vi "Main.vi"() -> ()   [LabVIEW 2022 SP3]
doc: "This Continuous Measurement sample project is based on the Queued Message Handler template.\n\nThe Event Handling Loop generates messages based on user interface actions.\n\nThe Message Handling Loop processes messages generated by the Event Handling Loop, or by other messages. There are also Acquisition and Logging message handling loop subVIs, and a chart updating loop."
uses:
  controls/UI State.ctl
  Settings/Settings.ctl
  Acquisition/Hardware Configuration.ctl
  Logging/Logging Configuration.ctl
  controls/UI Data.ctl
  <vilib>/Utility/miscctls.llb/LVMinMaxIncTypeDef.ctl
  <vilib>/Platform/browser.llb/Open URL in Default Browser (string).vi
  support/Message Queue/Enqueue Message (Array).vi
  <vilib>/Utility/error.llb/Error Cluster From Error Code.vi
  <vilib>/ErrorRing/Error Ring.xnode
  Acquisition/Acquisition.lvlib
  Logging/Logging.lvlib
  Settings/Settings.lvlib
  support/User Event - Stop/User Event - Stop.lvlib
  support/Message Queue/Message Queue.lvlib
  <instrlib>/BK Precision 911X Series/BK Precision 911X Series.lvlib
  Settings/Settings Dialog.vi
  Settings/Logging Settings Dialog.vi
  Settings/PS Settings Dialog.vi
  About.vi
panel:
  out "UI State":T1
  out "List CtlRef":refnum<vi>
  out "Settings CtlRef":refnum<vi>
  out "Output Ref":refnum<vi>
  in  "Clear":bool
  out "Stop":i32
  out "Power":dbl format="%.3g"
  out "Current":dbl format="%.3g"
  out "Voltage":dbl format="%.3g"
  out "model":string
  in  "PS Settings":bool
  in  "Tab Control":enum32{"Monitoring", "List", "Ext.Program"}(tab)
  out "Voltage":dbl(graph)
  out "Power":dbl(graph)
  out "Current":dbl(graph)
  in  "Keep Output Enable":bool
  in  "Enable Logging":bool
  in  "Abort List":bool
  in  "Run List":bool
  in  "List Array":T2(array[cluster]) {"Voltage" min=0.0 max=150.0 step=1.0 format="%.3g"; "Slope" min=0.0 max=30.0 step=1.0 format="%.3g"; "Current" format="%.3g"; "Width" min=0.001 max=86400.0 step=1.0 format="%.3g"}
  in  "List Number":i32=1
  in  "Sequence Number":dbl=1.0
  in  "Save List to PS":bool
  in  "Load List from PS":bool
  in  "List Power Limit":dbl
  in  "Sequence Repeat Count":i32[](array[numeric])
  in  "Linked Sequences":bool[](array[boolean])
  in  "Save Sequence to PS":bool
  in  "Load Sequence from PS":bool
  in  "List Repeat":i32=1 min=1 max=65535 step=1
  in  "Active Steps":bool[](array[boolean])
  out "Delay Time":dbl caption="Elapsed Time (s)"
  out "Elapsed Time (s)":dbl
  out "Start Time":string
  out "Stop Time":string
  out "Current Step":i32
  out "Remaining Steps":i32
  in  "Ext. List Abort":bool
  in  "Ext. List Start":bool
  in  "List Repeat":i32=1 min=1 step=1
  in  "Ext. List Array":T3(array[cluster]) {"Ext. List Voltage" min=0.0 max=150.0 step=1.0 format="%.3g"; "Ext. List Current" min=0.0 max=30.0 step=1.0 format="%.3g"; "Ext. List Time" min=0.001 max=86400.0 format="%.3g"}
  in  "Log Settings":bool
  in  "Meas Out":T4={"Voltage"=0.0, "Current"=0.0, "Power"=0.0, timestamp(3748437232.444618 s since 1904-01-01)}
  in  "Disconnect":bool
  in  "Output Control":bool
  out "ID":string="BK PRECISION, BK9116, 602078010687320001, 0.05-0.02\n"
  in  "Connect":bool
  in  "Inst. Settings":bool
  in  "Current":dbl(knob) min=0.0 max=30.0 step=1.0 scale=0.0..30.0 scale format="%#_3p"
  in  "Voltage":dbl(knob) min=0.0 max=150.0 step=1.0 scale=0.0..150.0 scale format="%#_2p"
  in  "Start":bool
  in  "Stop":bool
  out "Status":string="Exit"
  in  "Exit":bool
  # "Sequence Setup"
  # "List Setup"
  # "Step \nIndex"
  # "Voltage (V)"
  # "Current (A)"
  # "Time (s)"
  # "Output"
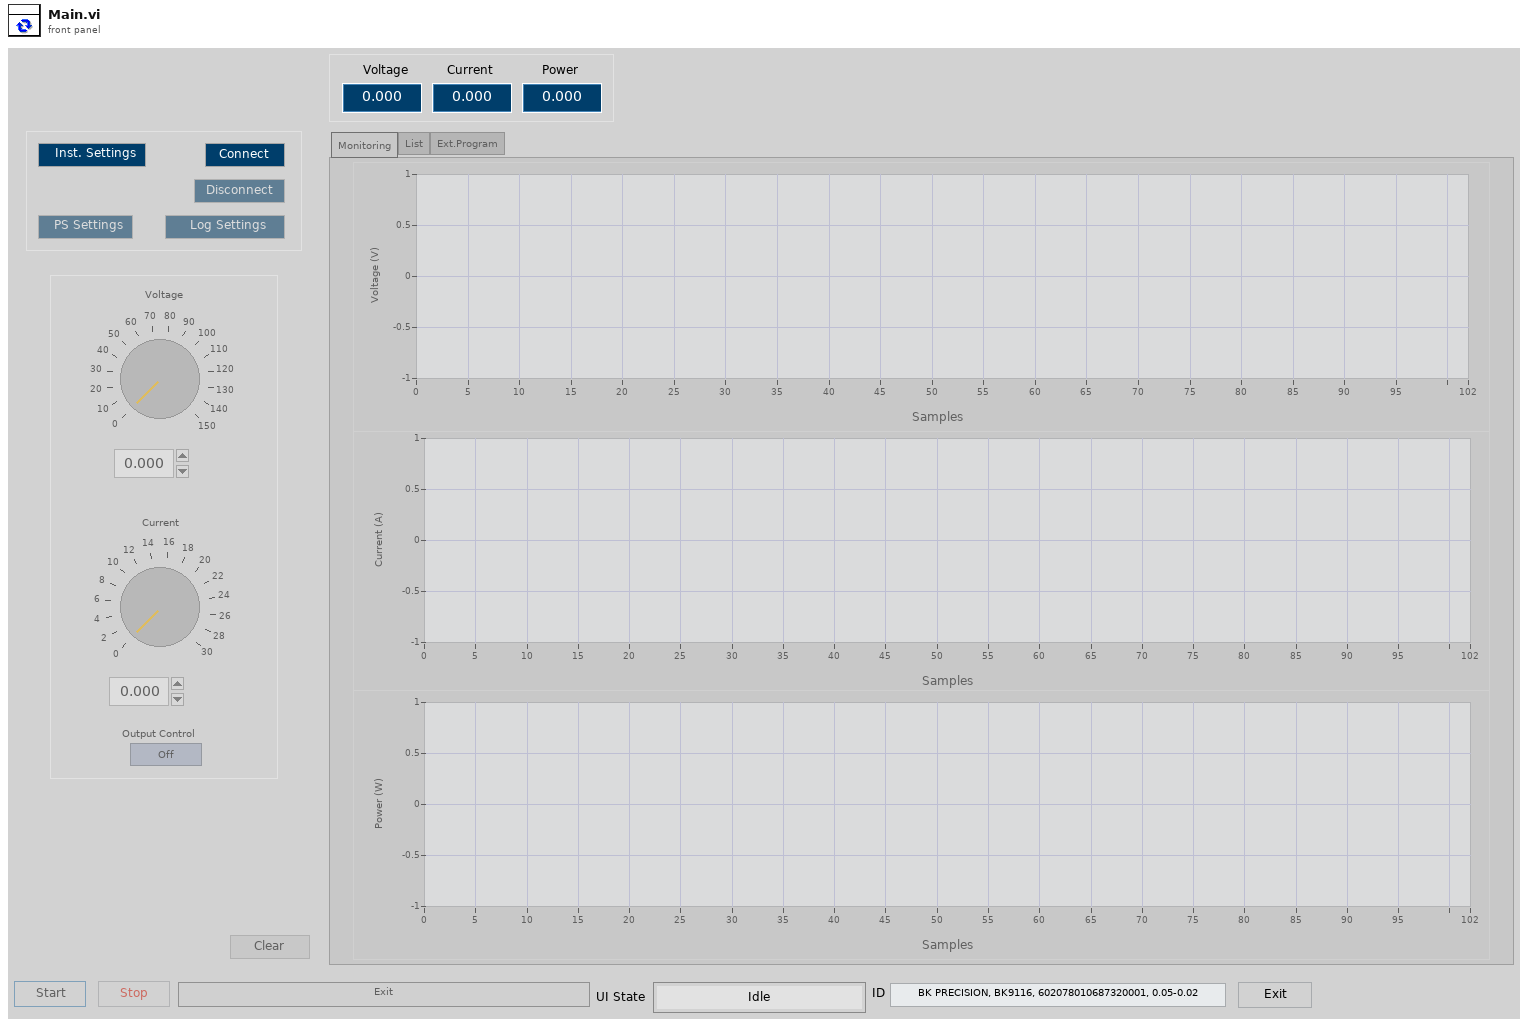
[diagram p1: front panel]
types:
  T1 = typedef "UI State.ctl" = enum16{"Idle", "Acquiring and Logging", "Waiting for Exit", "Waiting for Exit (Acq Stopped)", "Waiting for Exit (Log Stopped)", "Waiting for Stop", "Waiting for Stop (Acq Stopped)", "Waiting for Stop (Log Stopped)"}
  T2 = cluster{"Width":dbl, "Current":dbl, "Slope":dbl, "Voltage":dbl}[]
  T3 = cluster{"Boolean":bool, "Ext. List Time":dbl, "Ext. List Current":dbl, "Ext. List Voltage ":dbl}[]
  T4 = cluster{"Voltage":dbl, "Current":dbl, "Power":dbl, timestamp}
  T5 = cluster{"List Stop COND":i32, "Voltage":dbl, "Current":dbl, "Power":dbl}
  T6 = typedef "UI Data.ctl" = cluster{"Start Ref":refnum<vi>, "Stop Ref":refnum<vi>, "Connect Ref":refnum<vi>, "Exit Ref":refnum<vi>, "Status Ref":refnum<vi>, "Voltage":refnum<vi>, "Current":refnum<vi>, "Output Control":refnum<vi>, "TabCtl Refnum":refnum<vi>, "Inst.Settings Refnum":refnum<vi>, "PS Settings Refnum":refnum<vi>, "Log Settings Refnum":refnum<vi>, "Clear Refnum":refnum<vi>, "Disconnect Ref":refnum<vi>, "Run List Ref":refnum<vi>, "Abort List Ref":refnum<vi>}
  T7 = typedef "Settings.lvlib/Settings.ctl" = cluster{"Hardware Configuration":T8, "Logging Configuration":T9, "OVP Limit":dbl, "Current Limit":dbl, "OVP State":bool, "OVP Delay":dbl, "Voltage Limit":cluster{"Numeric":dbl, "Numeric":dbl}}
  T8 = typedef "Acquisition.lvlib/Hardware Configuration.ctl" = cluster{"VISA resource name":refnum<visa-resource-name>, "Baud Rate":u32, "Reset on Connect":bool, "Log Interval (s)":dbl, "Voltage":refnum<vi>, "Current":refnum<vi>, "Output Control":refnum<vi>}
  T9 = typedef "Logging.lvlib/Logging Configuration.ctl" = cluster{"Log File Base Path":path, "*IDN?":string, "File Path Ref":refnum<file>, "Log Interval (s)":dbl, "Enable TimeStamp":bool, "Append File":bool}
  T10 = typedef "Message Queue.lvlib/All Message Queues.ctl" = cluster{"UI":refnum<queue>, "Acquisition":refnum<queue>, "Logging":refnum<queue>}
  T11 = enum8{"Enabled", "Disabled", "Disabled and Grayed Out"}
  T12 = typedef "LVMinMaxIncTypeDef.ctl" = cluster{"Minimum":dbl, "Maximum":dbl, "Increment":dbl}
  T13 = cluster{"Ext. List Time 2":dbl, "Ext. List Time":dbl, "Ext. List Current":dbl, "Ext. List Voltage ":dbl}[]
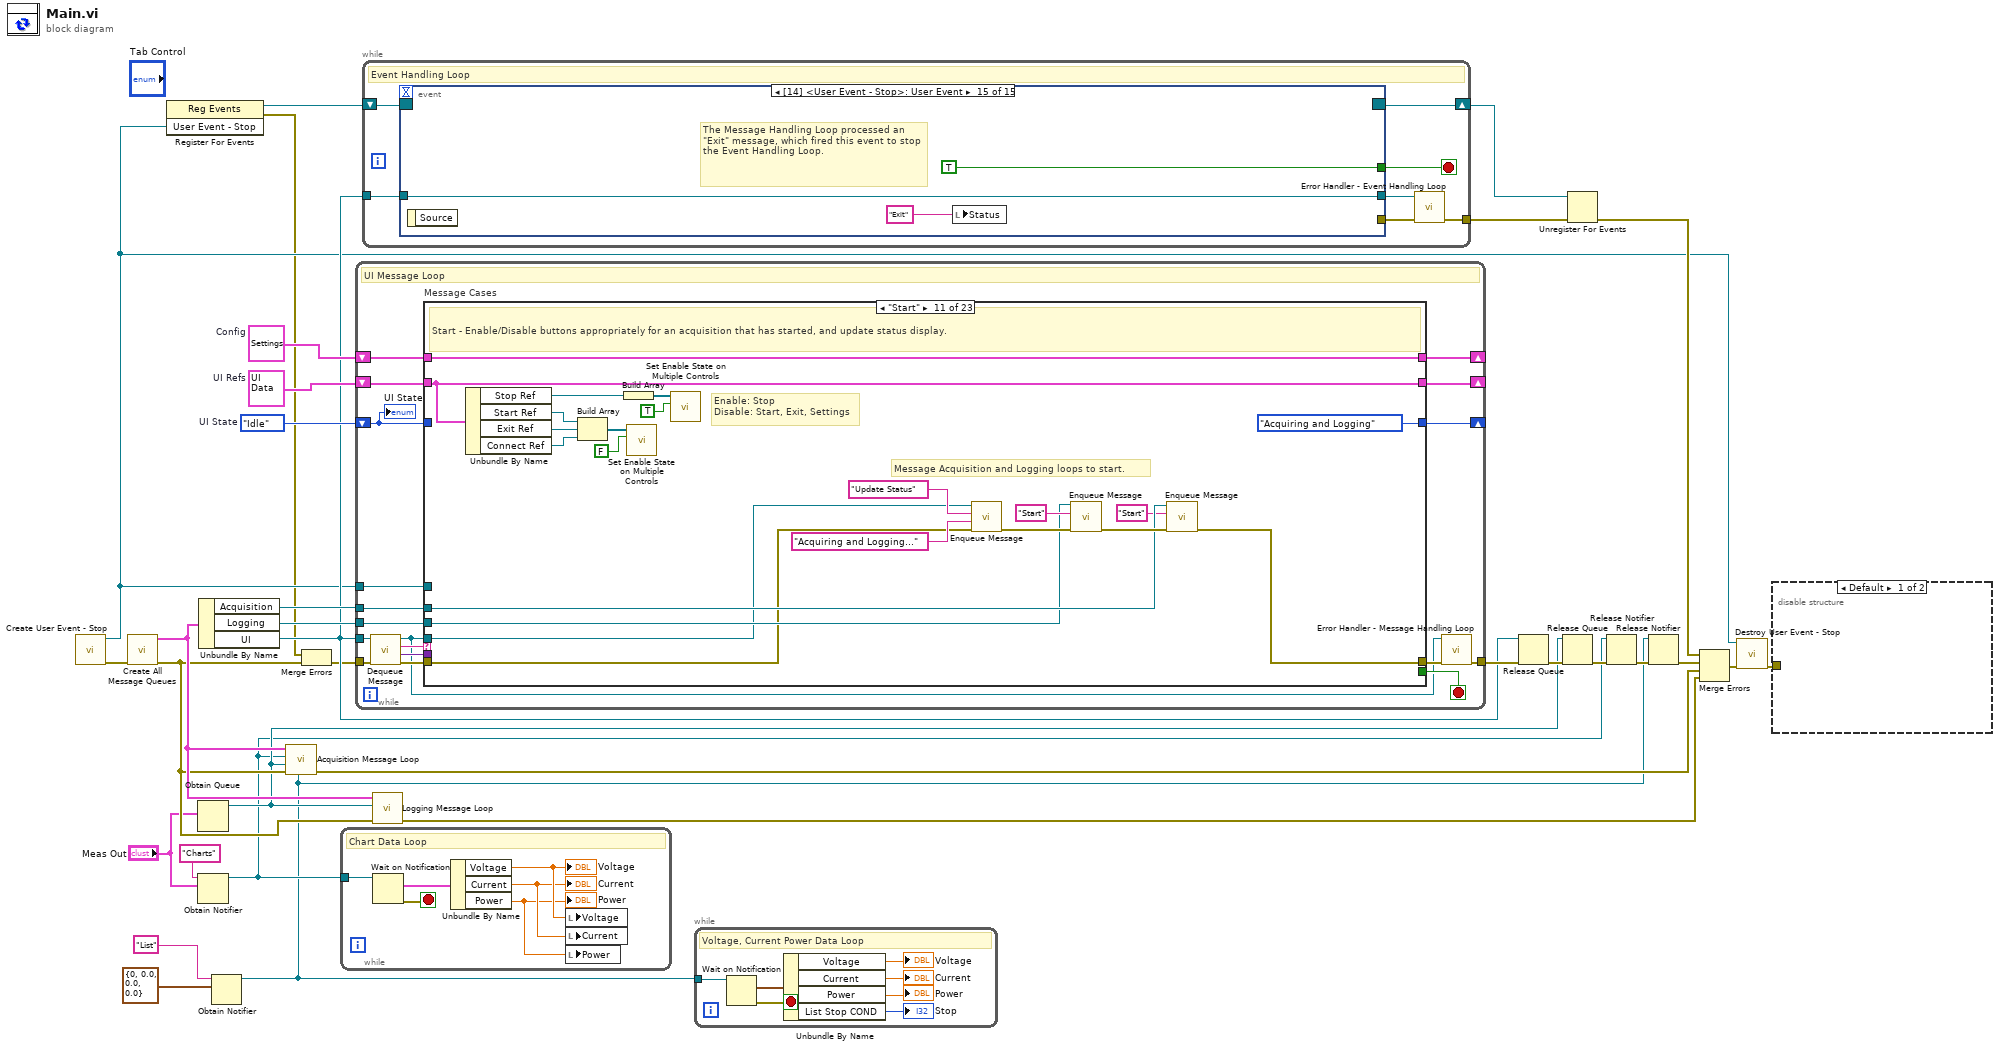
[diagram p0: block diagram]
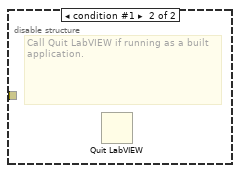
[diagram p2: hidden frame]
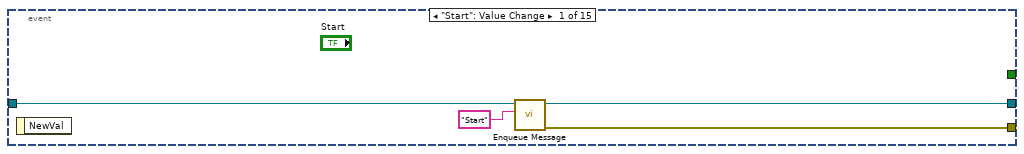
[diagram p3: hidden frame]
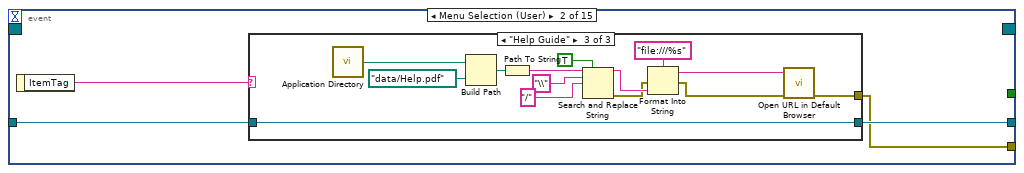
[diagram p4: hidden frame]
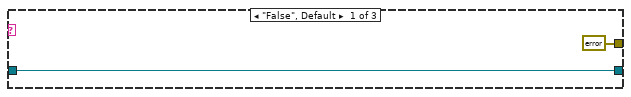
[diagram p5: hidden frame]
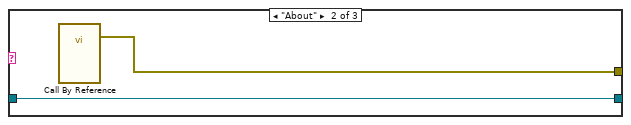
[diagram p6: hidden frame]
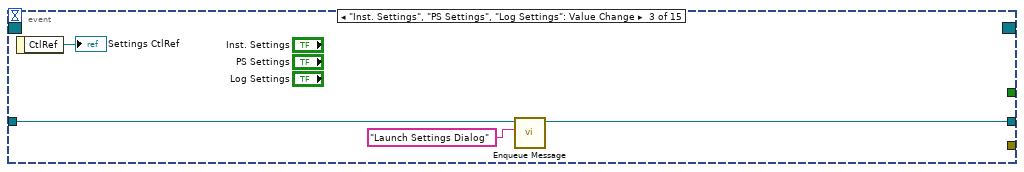
[diagram p7: hidden frame]
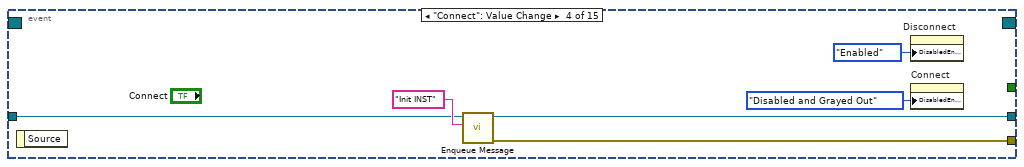
[diagram p8: hidden frame]
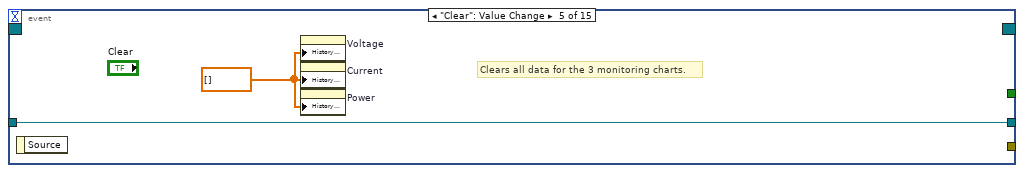
[diagram p9: hidden frame]
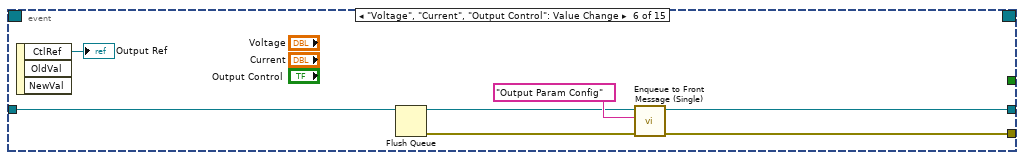
[diagram p10: hidden frame]
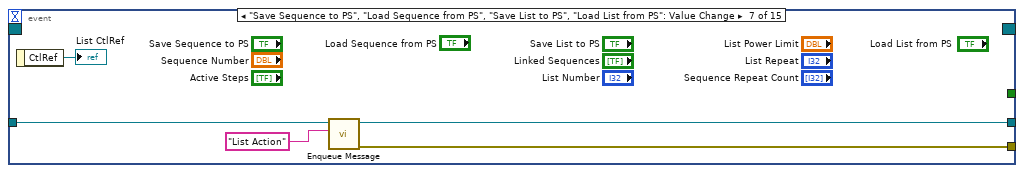
[diagram p11: hidden frame]
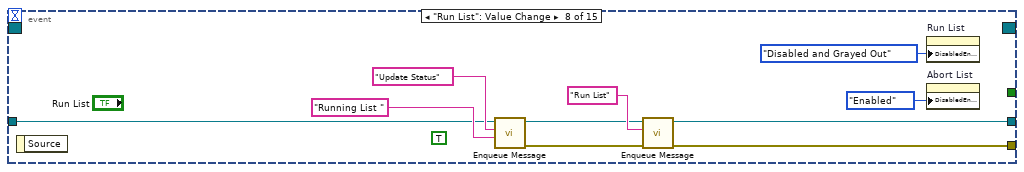
[diagram p12: hidden frame]
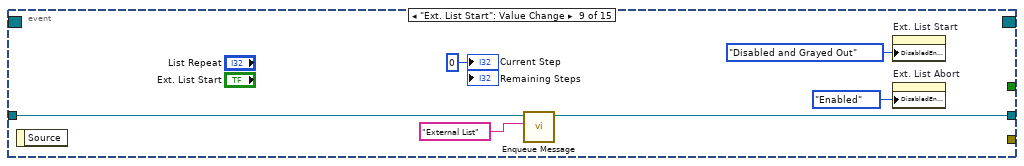
[diagram p13: hidden frame]
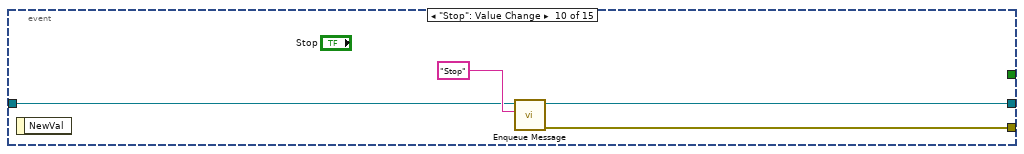
[diagram p14: hidden frame]
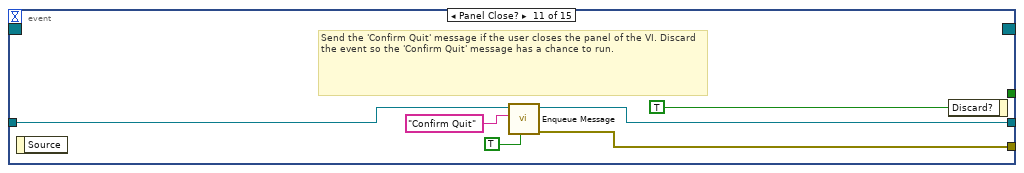
[diagram p15: hidden frame]
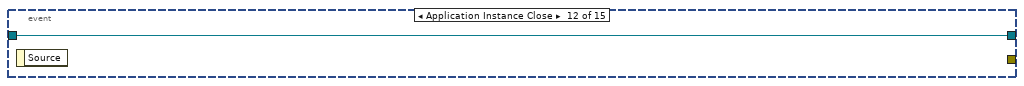
[diagram p16: hidden frame]
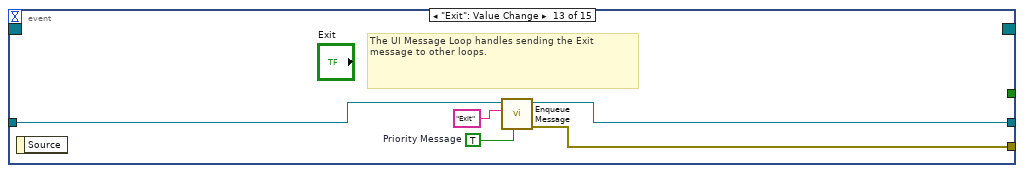
[diagram p17: hidden frame]
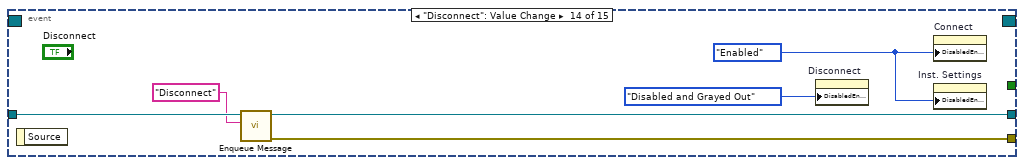
[diagram p18: hidden frame]
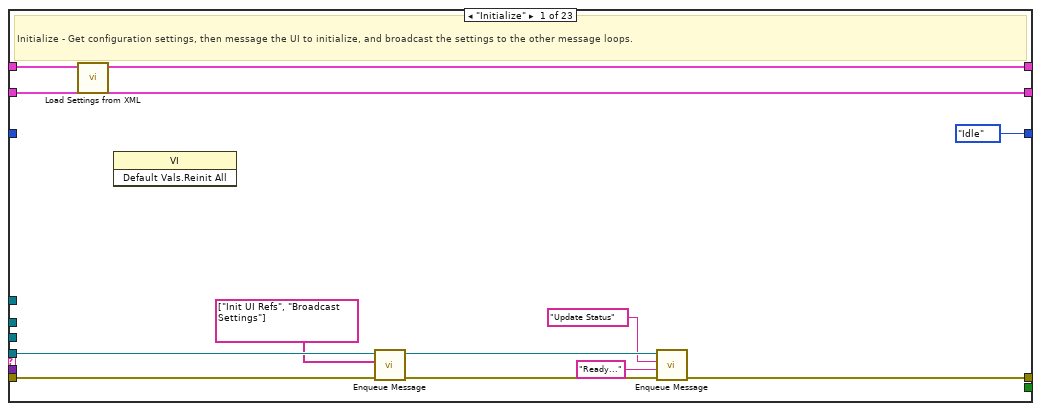
[diagram p19: hidden frame]
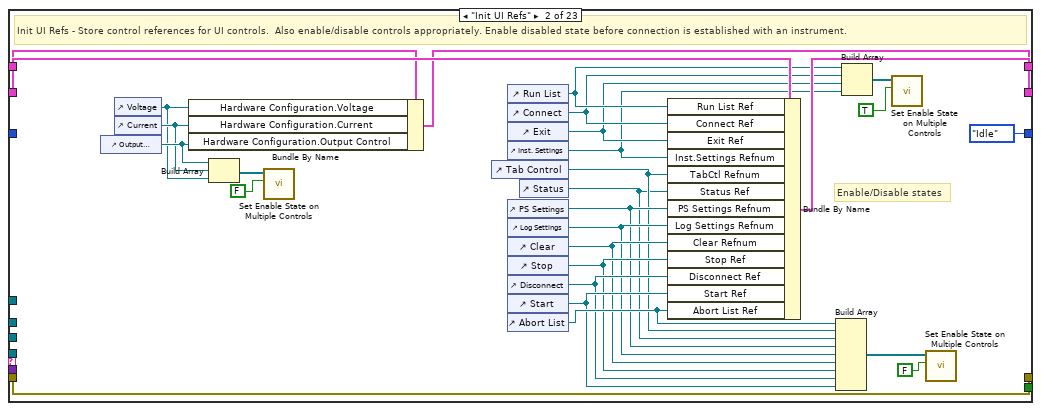
[diagram p20: hidden frame]
diagram:
  w19 = UI_State."Idle"  # UI State
  w22 = T6 {"Start Ref"=refnum, "Stop Ref"=refnum, "Connect Ref"=refnum, "Exit Ref"=refnum, "Status Ref"=refnum, "Voltage"=refnum, "Current"=refnum, "Output Control"=refnum, "TabCtl Refnum"=refnum, "Inst.Settings Refnum"=refnum, "PS Settings Refnum"=refnum, "Log Settings Refnum"=refnum, "Clear Refnum"=refnum, "Disconnect Ref"=refnum, "Run List Ref"=refnum, "Abort List Ref"=refnum}  # UI Refs
  w25 = T7 {"Hardware Configuration"={"VISA resource name"="", "Baud Rate"=0, "Reset on Connect"=FALSE, "Log Interval (s)"=0.0, "Voltage"=refnum, "Current"=refnum, "Output Control"=refnum}, "Logging Configuration"={"Log File Base Path"=path "", "*IDN?"="", "File Path Ref"=refnum, "Log Interval (s)"=0.0, "Enable TimeStamp"=FALSE, "Append File"=FALSE}, "OVP Limit"=0.0, "Current Limit"=0.0, "OVP State"=FALSE, "OVP Delay"=0.0, "Voltage Limit"={"Numeric"=0.0, "Numeric"=0.0}}  # Config
  n1 = call "Create User Event - Stop.vi"() -> ("error out"=w29:errorcluster, "User Event - Stop"=w12:refnum<user-event>)  [unwired: 10 in]
  n2 = call "Create All Message Queues.vi"("error in (no error)"=w29) -> ("error out"=w26:errorcluster, "Message Queues out"=w28:T10)  [unwired: 9 in]
  n3 = register-events(w12) -> (reference out=w13:refnum<event-registration>, error out=w10:errorcluster)  [unwired: 2 in]
  n4 = Obtain Queue(element data type="Meas Out") -> (queue out=w9:refnum<queue>)  [unwired: 4 in, 2 out]
  n5 = Obtain Notifier(name (unnamed)="Charts", notification data type="Meas Out") -> (notifier out=w2:refnum<notifier>)  [unwired: 2 in, 2 out]
  n6 = Unbundle By Name(w28) -> ("Acquisition"=w21:refnum<queue>, "Logging"=w20:refnum<queue>, "UI"=w17:refnum<queue>)
  n7 = Obtain Notifier(name (unnamed)="List", notification data type=T5 {"List Stop COND"=0, "Voltage"=0.0, "Current"=0.0, "Power"=0.0} ("List Data Out")) -> (notifier out=w1:refnum<notifier>)  [unwired: 2 in, 2 out]
  n8 = call "Acquisition Message Loop.vi"("List Notifier"=w1, "error in (no error)"=w26, "Data Queue"=w9, "Data Notifier"=w2, "Message Queues"=w28) -> ("error out"=w30:errorcluster)  [unwired: 6 in]
  n9 = Merge Errors(w10, w26) -> (w11:errorcluster)
  n10 = while "Data Display Loop" {
    tunnel: w2 -> [w38]
    stop <- w37 stop-if-true
    # "Chart Data Loop"
    n11 = Wait on Notification(notifier=w38) -> (notification=w36:T4, error out=w37:errorcluster)  [unwired: 3 in, 2 out]
    n12 = Unbundle By Name(w36) -> ("Voltage"=w35:dbl, "Current"=w34:dbl, "Power"=w33:dbl)
    "Voltage" <- w35
    "Power" <- w33
    "Current" <- w34
    n13 = local write "Voltage"(w35) -> ()
    n14 = local write "Current"(w34) -> ()
    n15 = local write "Power"(w33) -> ()
  }
  n16 = while {
    tunnel: w17 -> [w50]
    tunnel: w12 -> [w55]
    shift-right: [w49] -> _
    shift-left: w25 -> [w48]
    shift-right: [w46] -> _
    shift-left: w22 -> [w47]
    tunnel: w21 -> [w45]
    tunnel: w20 -> [w44]
    shift-right: [w40] -> _
    shift-left: w19 -> [w39]
    tunnel: w11 -> [w54]
    tunnel: [w43] -> w32
    stop <- w56 stop-if-true
    # "UI Message Loop"
    n17 = call "Dequeue Message.vi"("error in (no error)"=w54, "Message Queue"=w50) -> ("error out"=w53:errorcluster, "Message Data"=w51:variant, "Message"=w52:string, "dup Message Queue"=w41:refnum<queue>)  [unwired: 6 in]
    n18 = case "Message Cases" shown="\"Start\"" w52 {
      selector: w52 -> [_ _ _ _ _ _ _ _ _ _ _ _ _ _ _ _ _ _ _ _ _ _ w765]
      tunnel: w41 -> [w61 _ w111 _ _ _ _ w218 w353 w438 w519 _ w564 w589 _ w627 _ _ w709 w735 _ _ _]
      tunnel: w53 -> [w60 w95 w103 w120 w159 w167 w176 w229 w355 w441 w518 w540 w565 w590 w618 w632 w688 w698 w708 w737 w746 w763 _]
      tunnel: [w65 w95 w106 w119 w159 w164 w177 w230 w352 w440 w524 w543 w562 w587 w612 w629 w689 w702 w707 w740 w756 w762 w764] -> w42
      tunnel: [_ _ _ _ _ _ _ _ _ _ _ _ _ _ _ _ _ _ _ _ TRUE _ _] -> w56
      tunnel: w51 -> [_ _ _ w122 _ w166 _ _ _ _ _ _ _ _ _ _ _ w701 _ _ w744 _ _]
      tunnel: w55 -> [_ _ _ _ _ _ _ _ _ _ _ _ _ _ _ _ _ _ _ _ w757 _ _]
      tunnel: [w68 w89 w115 w117 w147 w162 w174 w234 w358 w443 w539 w559 w568 w593 w622 w624 w696 w705 w712 w739 w755 w761 w768] -> w49
      tunnel: w48 -> [w57 w90 w105 w117 w147 w162 w174 w234 w358 w443 w539 w559 w568 w593 w622 w625 w696 w705 w712 w739 w755 w761 w768]
      tunnel: w47 -> [w62 w94 w116 w118 w148 w161 w178 w235 w359 w444 w536 w558 w567 w592 w616 w631 w697 w704 w711 w742 w754 w760 w767]
      tunnel: [w62 w93 w116 w118 w148 w161 w178 w235 w359 w444 w536 w558 w567 w592 w616 w631 w697 w704 w711 w742 w754 w760 w767] -> w46
      tunnel: w45 -> [_ _ _ _ _ _ w170 w219 w354 w437 w523 w548 _ _ w615 _ _ _ _ _ w753 _ _]
      tunnel: w44 -> [_ _ _ _ _ _ _ _ w350 _ w520 w541 _ _ w614 _ _ _ _ _ w752 _ _]
      tunnel: w39 -> [_ _ _ _ _ w160 w175 w220 w357 w439 _ w545 w566 w591 w613 w630 _ w700 w710 _ _ w759 w766]
      tunnel: [UI_State."Idle" ("UI State") UI_State."Idle" ("UI State") UI_State."Idle" ("UI State") UI_State."Idle" ("UI State") UI_State."Idle" ("UI State") w160 w168 UI_State."Idle" ("UI State") w351 w442 UI_State."Acquiring and Logging" ("UI State") w546 w563 w588 w613 w630 UI_State."Idle" ("UI State") w700 w706 UI_State."Idle" ("UI State") UI_State."Idle" ("UI State") w759 w766] -> w40
      frame "Initialize" {
        # "Initialize - Get configuration settings, then message the UI to initialize, and broadcast the settings to the other message loops."
        n19 = call "Load Settings from XML.vi"("Settings in"=w57) -> ("Settings out"=w68:T7)  [unwired: 9 in, 1 out]
        n20 = invoke class="VI" method="Default Vals.Reinit All"() -> ()  [unwired: 3 in, 3 out]
        n21 = call-poly "Enqueue Message.vi"("error in (no error)"=w60, "Message Array"=string[] ["Init UI Refs", "Broadcast Settings"], "Message Queue"=w61) -> ("error out"=w67:errorcluster, "dup Message Queue"=w66:refnum<queue>)  [unwired: 7 in]
        n22 = call-poly "Enqueue Message.vi"("error in (no error)"=w67, "Message Data"="Ready..." ("Ready..."), "Message"="Update Status", "Message Queue"=w66) -> ("error out"=w65:errorcluster)  [unwired: 6 in, 1 out]
      }
      frame "Init UI Refs" {
        # "Enable/Disable states"
        # "Init UI Refs - Store control references for UI controls.  Also enable/disable controls appropriately. Enable disabled state before connection is established with an instrument."
        n23 = control-ref of="Output Control"() -> (w73:refnum<vi>)
        n24 = control-ref of="Voltage"() -> (w71:refnum<vi>)
        n25 = control-ref of="Current"() -> (w72:refnum<vi>)
        n26 = Bundle By Name(cluster=w90, "Hardware Configuration.Voltage"=w71, "Hardware Configuration.Current"=w72, "Hardware Configuration.Output Control"=w73) -> (w89:T7)
        n27 = Build Array(w73, w72, w71) -> (w70:refnum<vi>[])
        n28 = call "Set Enable State on Multiple Controls.vi"("Enable?"=FALSE, "Controls"=w70) -> ()  [unwired: 10 in]
        n29 = control-ref of="Tab Control"() -> (w80:refnum<vi>)
        n30 = control-ref of="Run List"() -> (w77:refnum<vi>)
        n31 = control-ref of="Connect"() -> (w76:refnum<vi>)
        n32 = control-ref of="Exit"() -> (w75:refnum<vi>)
        n33 = control-ref of="Inst. Settings"() -> (w74:refnum<vi>)
        n34 = control-ref of="PS Settings"() -> (w81:refnum<vi>)
        n35 = control-ref of="Log Settings"() -> (w82:refnum<vi>)
        n36 = control-ref of="Clear"() -> (w83:refnum<vi>)
        n37 = control-ref of="Stop"() -> (w84:refnum<vi>)
        n38 = control-ref of="Disconnect"() -> (w85:refnum<vi>)
        n39 = control-ref of="Start"() -> (w86:refnum<vi>)
        n40 = control-ref of="Abort List"() -> (w96:refnum<vi>)
        n41 = control-ref of="Status"() -> (w78:refnum<vi>)
        n42 = Bundle By Name(cluster=w94, "Run List Ref"=w77, "Connect Ref"=w76, "Exit Ref"=w75, "Inst.Settings Refnum"=w74, "TabCtl Refnum"=w80, "Status Ref"=w78, "PS Settings Refnum"=w81, "Log Settings Refnum"=w82, "Clear Refnum"=w83, "Stop Ref"=w84, "Disconnect Ref"=w85, "Start Ref"=w86, "Abort List Ref"=w96) -> (w93:T6)
        n43 = Build Array(w96, w80, w78, w81, w82, w83, w84, w85, w86) -> (w79:refnum<vi>[])
        n44 = Build Array(w77, w76, w75, w74) -> (w88:refnum<vi>[])
        n45 = call "Set Enable State on Multiple Controls.vi"("Enable?"=TRUE, "Controls"=w88) -> ()  [unwired: 10 in]
        n46 = call "Set Enable State on Multiple Controls.vi"("Enable?"=FALSE, "Controls"=w79) -> ()  [unwired: 10 in]
      }
      frame "Init INST" {
        # "Connect instrument and get identification string. Parse model number from identification string and proceed to Configure UI and Update enable/disable states."
        n47 = Unbundle By Name(w105) -> ("Hardware Configuration.Baud Rate"=w99:u32, "Hardware Configuration.VISA resource name"=w100:refnum<visa-resource-name>, "Hardware Configuration.Reset on Connect"=w98:bool)
        n48 = call "Initialize.vi"("Baud Rate"=w99, "error in (no error)"=w103, "ID Query (True)"=TRUE, "Reset (True)"=w98, "VISA resource name"=w100) -> ("error out"=w102:errorcluster, "*IDN?"=w101:string)  [unwired: 4 in, 1 out]
        "ID" <- w101
        n49 = String Subset(string=w101, offset (0)=16, length (rest)=4 ("length (rest)")) -> (substring=w109:string)
        "model" <- w109
        n50 = call "Enqueue Message (Single).vi"("error in (no error)"=w102, "Message Data"=w109, "Message"="Config UI", "Message Queue"=w111) -> ("error out"=w107:errorcluster, "dup Message Queue"=w108:refnum<queue>)  [unwired: 6 in]
        n51 = Bundle By Name(cluster=w105, "Logging Configuration.*IDN?"=w101) -> (w115:T7)
        n52 = call "Enqueue Message (Single).vi"("error in (no error)"=w107, "Message"="UI REF Connection Update", "Message Queue"=w108) -> ("error out"=w106:errorcluster)  [unwired: 7 in, 1 out]
      }
      frame "Config UI" {
        # "Configure the UI limits based on the model number of the instrument connected."
        n53 = Variant To Data(type="", Variant=w122) -> (data=w121:string)  [unwired: 1 in, 1 out]
        n54 = case shown="\"9116\"" w121 {
          tunnel: w120 -> [w125 w128 w133]
          tunnel: [w125 w128 w133] -> w119
          tunnel: w117 -> [_ _ _]
          frame "False", Default {
          }
          frame "9115" {
            w127 = T12 {"Minimum"=0.0, "Maximum"=80.0, "Increment"=1.0} ("Data Entry Limits")
            w126 = T12 {"Minimum"=0.0, "Maximum"=60.0, "Increment"=1.0} ("Data Entry Limits")
            n55 = property on="Ext. List Voltage" class="DigNum (strict)"("Data Range"=w127) -> ()  [unwired: 2 in, 2 out]
            n56 = property on="Voltage" class="Knob (strict)"("Data Range"=w127, "Scale.Maximum"=80.0 ("Scale.Range:Maximum")) -> ()  [unwired: 2 in, 2 out]
            n57 = property on="Ext. List Current" class="DigNum (strict)"("Data Range"=w126) -> ()  [unwired: 2 in, 2 out]
            n58 = property on="Current" class="Knob (strict)"("Data Range"=w126, "Scale.Maximum"=60.0 ("Scale.Range:Maximum")) -> ()  [unwired: 2 in, 2 out]
            n59 = property on="Voltage" class="DigNum (strict)"("Data Range"=w127) -> ()  [unwired: 2 in, 2 out]
            n60 = property on="Slope" class="DigNum (strict)"("Data Range"=w126) -> ()  [unwired: 2 in, 2 out]
          }
          frame "9116" {
            w131 = T12 {"Minimum"=0.0, "Maximum"=150.0, "Increment"=1.0} ("Data Entry Limits")
            w132 = T12 {"Minimum"=0.0, "Maximum"=30.0, "Increment"=1.0} ("Data Entry Limits")
            n61 = property on="Ext. List Voltage" class="DigNum (strict)"("Data Range"=w131) -> ()  [unwired: 2 in, 2 out]
            n62 = property on="Voltage" class="Knob (strict)"("Data Range"=w131, "Scale.Maximum"=150.0 ("Scale.Range:Maximum")) -> ()  [unwired: 2 in, 2 out]
            n63 = property on="Ext. List Current" class="DigNum (strict)"("Data Range"=w132) -> ()  [unwired: 2 in, 2 out]
            n64 = property on="Current" class="Knob (strict)"("Data Range"=w132, "Scale.Maximum"=30.0 ("Scale.Range:Maximum")) -> ()  [unwired: 2 in, 2 out]
            n65 = property on="Voltage" class="DigNum (strict)"("Data Range"=w131) -> ()  [unwired: 2 in, 2 out]
            n66 = property on="Slope" class="DigNum (strict)"("Data Range"=w132) -> ()  [unwired: 2 in, 2 out]
          }
        }
      }
      frame "UI REF Connection Update" {
        # "Enable: States"
        # "Disable: States"
        # "Enable: States"
        # "UI Refs Update- Enable/disable controls appropriately. Enable disabled state after connection is established with an instrument."
        n67 = Unbundle By Name(w147) -> ("Hardware Configuration.Voltage"=w151:refnum<vi>, "Hardware Configuration.Current"=w150:refnum<vi>, "Hardware Configuration.Output Control"=w149:refnum<vi>)
        n68 = Unbundle By Name(w148) -> ("Connect Ref"=w145:refnum<vi>, "Stop Ref"=w146:refnum<vi>, "Inst.Settings Refnum"=w144:refnum<vi>, "TabCtl Refnum"=w139:refnum<vi>, "Status Ref"=w140:refnum<vi>, "PS Settings Refnum"=w141:refnum<vi>, "Log Settings Refnum"=w143:refnum<vi>, "Clear Refnum"=w142:refnum<vi>, "Exit Ref"=w136:refnum<vi>, "Disconnect Ref"=w137:refnum<vi>, "Start Ref"=w138:refnum<vi>)
        n69 = Build Array(w145, w146, w144) -> (w156:refnum<vi>[])
        n70 = Build Array(w139, w140, w141, w143, w142, w136, w137, w138) -> (w154:refnum<vi>[])
        n71 = call "Set Enable State on Multiple Controls.vi"("Enable?"=FALSE, "Controls"=w156) -> ()  [unwired: 10 in]
        n72 = Build Array(w151, w150, w149) -> (w153:refnum<vi>[])
        n73 = call "Set Enable State on Multiple Controls.vi"("Enable?"=TRUE, "Controls"=w154) -> ()  [unwired: 10 in]
        n74 = call "Set Enable State on Multiple Controls.vi"("Enable?"=TRUE, "Controls"=w153) -> ()  [unwired: 10 in]
      }
      frame "Update Status" {
        # "Update Status - Convert the message data to a string to display in the Status indicator."
        n75 = Variant To Data(error in=w167, type="", Variant=w166) -> (data=→"Status":string, error out=w164:errorcluster)
      }
      frame "Output Param Config" {
        # "Configure the modified parameter of the output. (Voltage, Current, or State) If UI State is acquiring and logging this function is instead performed in the Acquisition Message loop to prevent timeout errors with the main vi and the Acquisition Message Loop vi. Note that the parameter configuration will have priority over acquisition queue."
        n76 = Unbundle By Name(w174) -> ("Hardware Configuration.VISA resource name"=w171:refnum<visa-resource-name>)
        n77 = local read "Output Ref"() -> (w173:refnum<vi>)
        n78 = property on="Property Node" class="Ctl"(reference=w173) -> (reference out=w169:refnum<vi>, "Label.Text"=w172:string)  [unwired: 1 in, 1 out]
        n79 = case shown="\"Idle\", Default" w175 {
          tunnel: [w180 w200] -> w177
          tunnel: w176 -> [w181 w201]
          tunnel: w172 -> [w183 w199]
          tunnel: w171 -> [w182 _]
          tunnel: w170 -> [_ w198]
          tunnel: w169 -> [_ _]
          tunnel: [w179 w197] -> w168
          frame "Idle", Default {
            w179 = UI_State."Idle"  # UI State
            n80 = case shown="\"False\", Default" w183 {
              tunnel: w182 -> [_ w187 w190 w194]
              tunnel: w181 -> [w184 w188 w191 w196]
              tunnel: [w184 w185 w192 w195] -> w180
              frame "False", Default {
              }
              frame "Voltage" {
                n81 = local read "Voltage"() -> (w186:dbl)
                n82 = call "Configure Voltage.vi"("Voltage"=w186, "error in (no error)"=w188, "VISA resource name"=w187) -> ("error out"=w185:errorcluster)  [unwired: 7 in, 1 out]
              }
              frame "Current" {
                n83 = local read "Current"() -> (w189:dbl)
                n84 = call "Configure Current.vi"("Current"=w189, "error in (no error)"=w191, "VISA resource name"=w190) -> ("error out"=w192:errorcluster)  [unwired: 7 in, 1 out]
              }
              frame "Output Control" {
                n85 = local read "Output Control"() -> (w193:bool)
                n86 = call <instrlib>:"Enable Output.vi"("error in (no error)"=w196, "Enable Output (F: False)"=w193, "VISA resource name"=w194) -> ("error out"=w195:errorcluster)  [unwired: 7 in, 1 out]
              }
            }
          }
          frame "Acquiring and Logging" {
            w197 = UI_State."Acquiring and Logging"  # UI State
            n87 = case shown="\"Output Control\"" w199 {
              selector: w199 -> [_ w204 w209 w214]
              tunnel: w201 -> [w202 w206 w211 w216]
              tunnel: [w202 w205 w210 w215] -> w200
              tunnel: w198 -> [_ w207 w212 w217]
              frame "False", Default {
              }
              frame "Voltage" {
                n88 = call-poly "Enqueue Message.vi"("Priority Message? (F)"=TRUE, "error in (no error)"=w206, "Message"=w204, "Message Queue"=w207) -> ("error out"=w205:errorcluster)  [unwired: 6 in, 1 out]
              }
              frame "Current" {
                n89 = call-poly "Enqueue Message.vi"("Priority Message? (F)"=TRUE, "error in (no error)"=w211, "Message"=w209, "Message Queue"=w212) -> ("error out"=w210:errorcluster)  [unwired: 6 in, 1 out]
              }
              frame "Output Control" {
                n90 = call-poly "Enqueue Message.vi"("Priority Message? (F)"=TRUE, "error in (no error)"=w216, "Message"=w214, "Message Queue"=w217) -> ("error out"=w215:errorcluster)  [unwired: 6 in, 1 out]
              }
            }
          }
        }
      }
      frame "List Action" {
        # "Save or Load a sequence or list's parameters. If UI state is Acquiring and Logging the acquisition will be terminated before completing the list action."
        n91 = Unbundle By Name(w234) -> ("Hardware Configuration.VISA resource name"=w233:refnum<visa-resource-name>)
        n92 = local read "List CtlRef"() -> (w221:refnum<vi>)
        n93 = local read "Sequence Repeat Count"() -> (w227:i32[])
        n94 = local read "Sequence Number"() -> (w232:dbl)
        n95 = local read "Linked Sequences"() -> (w226:bool[])
        n96 = local read "List Power Limit"() -> (w225:dbl)
        n97 = local read "List Number"() -> (w223:i32)
        n98 = local read "Active Steps"() -> (w231:bool[])
        n99 = local read "List Repeat"() -> (w224:i32)
        n100 = property on="Property Node" class="Bool"(reference=w221) -> ("Label.Text"=w222:string)  [unwired: 1 in, 2 out]
        n101 = case shown="\"Idle\", Default" w220 {
          tunnel: w233 -> [w247 _]
          tunnel: w232 -> [w246 _]
          tunnel: w231 -> [w245 _]
          tunnel: [w244 w346] -> w230
          tunnel: w229 -> [w243 w349]
          tunnel: w227 -> [w242 _]
          tunnel: w226 -> [w241 _]
          tunnel: w225 -> [w240 _]
          tunnel: w224 -> [w239 _]
          tunnel: w223 -> [w238 _]
          tunnel: w222 -> [w237 w339]
          tunnel: w219 -> [_ _]
          tunnel: w218 -> [w236 w344]
          frame "Idle", Default {
            n102 = case shown="\"Load Sequence from PS\"" w237 {
              selector: w237 -> [_ w253 w282 w296 w325]
              tunnel: w247 -> [_ w264 w293 w307 w329]
              tunnel: w246 -> [_ w263 w292 _ _]
              tunnel: w245 -> [_ w262 _ _ _]
              tunnel: [w248 w250 w284 w294 w327] -> w244
              tunnel: w243 -> [w248 w257 w291 w305 w332]
              tunnel: w242 -> [_ _ _ w306 w331]
              tunnel: w241 -> [_ _ _ w304 _]
              tunnel: w240 -> [_ _ _ w302 _]
              tunnel: w239 -> [_ _ _ w303 w330]
              tunnel: w238 -> [_ _ _ w301 _]
              tunnel: w236 -> [_ w252 w283 w297 w326]
              frame "False", Default {
              }
              frame "Save Sequence to PS" {
                # "Configure sequence's steps"
                # "Save sequence"
                # "Configure sequence"
                n103 = local read "List Array"() -> (w249:T2)
                n104 = call <instrlib>:"Configure Sequence.vi"("error in (no error)"=w257, "Active Steps (0000000000)"=w262, "Sequence Number (1)"=w263, "VISA resource name"=w264) -> ("error out"=w258:errorcluster, "VISA resource name out"=w261:refnum<visa-resource-name>)  [unwired: 6 in]
                n105 = for {
                  tunnel: w261 -> [w278]
                  tunnel: [w277] -> w260
                  tunnel: [w276] -> w259
                  tunnel: w258 -> [w275]
                  tunnel: w249 -> [w274] mode=indexing
                  i -> [w280]
                  n106 = Unbundle(w274) -> ("Width"=w270:dbl, "Current"=w271:dbl, "Slope"=w272:dbl, "Voltage"=w273:dbl)
                  n107 = Increment(x=w280) -> (x+1=w279:i32)
                  n108 = call "Configure Sequence Parameters.vi"("VISA resource name"=w278, "Step Number (1)"=w279, "Step Width (1)"=w270, "error in (no error)"=w275, "Step Current (1.000)"=w271, "Step Slope (1)"=w272, "Step Voltage (1.000)"=w273) -> ("VISA resource name out"=w277:refnum<visa-resource-name>, "error out"=w276:errorcluster)  [unwired: 7 in]
                }
                n109 = flat-sequence {
                  tunnel: w260 -> [w269]
                  tunnel: w259 -> [w268]
                  tunnel: [w267] -> _
                  tunnel: [w266] -> w251
                  frame #0 {
                    n110 = Wait (ms)(milliseconds to wait=u32 2000) -> ()  [unwired: 1 out]
                    n111 = call <instrlib>:"Save Sequence.vi"("error in (no error)"=w268, "VISA resource name"=w269) -> ("error out"=w266:errorcluster, "VISA resource name out"=w267:refnum<visa-resource-name>)  [unwired: 8 in]
                  }
                }
                n112 = Concatenate Strings(w253, " Complete" ("string")) -> (w255:string)
                n113 = call-poly "Enqueue Message.vi"("error in (no error)"=w251, "Message Data"=w255, "Message"="Update Status", "Message Queue"=w252) -> ("error out"=w250:errorcluster)  [unwired: 6 in, 1 out]
              }
              frame "Load Sequence from PS" {
                # "Load Sequence from PS"
                n114 = call "Read Sequence Data.vi"("error in"=w291, "Array"="List Array", "Sequence Number"=w292, "VISA resource name"=w293) -> ("error out"=w285:errorcluster, "Array Out"=w289:T13, "Actibve Steps"=w290:bool[])  [unwired: 4 in, 1 out]
                n115 = local write "Active Steps"(w290) -> ()
                n116 = local write "List Array"(w289) -> ()
                n117 = Concatenate Strings(w282, " Complete" ("string")) -> (w287:string)
                n118 = call-poly "Enqueue Message.vi"("error in (no error)"=w285, "Message Data"=w287, "Message"="Update Status", "Message Queue"=w283) -> ("error out"=w284:errorcluster)  [unwired: 6 in, 1 out]
              }
              frame "Save List to PS" {
                w309 = u16 0 items=["Save", "Recall"] ("Save Recall List File (0:Save)")
                # "Save List"
                # "Configure list"
                # "Configure List sequence repeat"
                n119 = call <instrlib>:"Configure List Parameters.vi"("VISA resource name"=w307, "List File Number (1)"=w301, "List Power Limit (1200)"=w302, "Repeat Count (1)"=w303, "Linked Sequences (0000000000)"=w304, "error in (no error)"=w305) -> ("VISA resource name out"=w314:refnum<visa-resource-name>, "error out"=w313:errorcluster)  [unwired: 8 in]
                n120 = for {
                  N: 10 -> [_]
                  tunnel: w314 -> [w321]
                  tunnel: w313 -> [w320]
                  tunnel: w306 -> [w319] mode=indexing
                  tunnel: [w316] -> w312
                  tunnel: [w315] -> w311
                  i -> [w318]
                  n121 = Increment(x=w318) -> (x+1=w317:i32)
                  n122 = call "Configure List Sequence Repeat.vi"("error in (no error)"=w320, "Repeat Count (1)"=w319, "Sequence Number (1)"=w317, "VISA resource name"=w321) -> ("error out"=w315:errorcluster, "VISA resource name out"=w316:refnum<visa-resource-name>)  [unwired: 6 in]
                }
                n123 = local read "List Number"() -> (w310:i32)
                n124 = call <instrlib>:"Save Recall List Program.vi"("error in (no error)"=w311, "List Number (1)"=w310, "Save Recall List File (0:Save)"=w309, "VISA resource name"=w312) -> ("error out"=w295:errorcluster)  [unwired: 6 in, 1 out]
                n125 = Concatenate Strings(w296, " Complete" ("string")) -> (w299:string)
                n126 = call-poly "Enqueue Message.vi"("error in (no error)"=w295, "Message Data"=w299, "Message"="Update Status", "Message Queue"=w297) -> ("error out"=w294:errorcluster)  [unwired: 6 in, 1 out]
              }
              frame "Load List from PS" {
                # "Load list's parameters from PS"
                n127 = call "Read List Data.vi"("Sequence Repeat Count"=w331, "error in"=w332, "List Number"=w330, "VISA resource name"=w329) -> ("error out"=w328:errorcluster, "List Repeat"=w335:i32, "Sequence Repeat Count Out"=w336:i32[], "Linked Sequences"=w333:bool[], "List Power Limit"=w334:dbl)  [unwired: 2 in, 1 out]
                n128 = local write "List Power Limit"(w334) -> ()
                n129 = local write "Sequence Repeat Count"(w336) -> ()
                n130 = local write "List Repeat"(w335) -> ()
                n131 = local write "Linked Sequences"(w333) -> ()
                n132 = Concatenate Strings(w325, " Complete" ("string")) -> (w323:string)
                n133 = call-poly "Enqueue Message.vi"("error in (no error)"=w328, "Message Data"=w323, "Message"="Update Status", "Message Queue"=w326) -> ("error out"=w327:errorcluster)  [unwired: 6 in, 1 out]
              }
            }
          }
          frame "Acquiring and Logging" {
            n134 = call-poly "Enqueue Message.vi"("Priority Message? (F)"=TRUE, "error in (no error)"=w349, "Message"="Stop", "Message Queue"=w344) -> ("error out"=w343:errorcluster, "dup Message Queue"=w342:refnum<queue>)  [unwired: 6 in]
            n135 = call-poly "Enqueue Message.vi"("error in (no error)"=w343, "Message Data"=w339, "Message"="Update Status", "Message Queue"=w342) -> ("error out"=w340:errorcluster, "dup Message Queue"=w341:refnum<queue>)  [unwired: 6 in]
            n136 = call-poly "Enqueue Message.vi"("error in (no error)"=w340, "Message"="List Action", "Message Queue"=w341) -> ("error out"=w346:errorcluster)  [unwired: 7 in, 1 out]
            n137 = One Button Dialog(message="Acquisition and Logging will stopped\nwhen completing a list or sequence action.") -> ()  [unwired: 1 in, 1 out]
          }
        }
      }
      frame "Run List" {
        # "Run the selected internal program. If UI state is Acquiring and Logging the acquisition will be terminated before completing the list action. Acquisition then begins on the List Acquisition case."
        n138 = Unbundle By Name(w358) -> ("Hardware Configuration.VISA resource name"=w356:refnum<visa-resource-name>)
        n139 = case shown="\"Idle\", Default" w357 {
          tunnel: w356 -> [w380 _]
          tunnel: w355 -> [w383 w430]
          tunnel: w354 -> [w382 w431]
          tunnel: w353 -> [w365 w426]
          tunnel: [w377 w428] -> w352
          tunnel: [UI_State."Idle" ("UI State") UI_State."Idle" ("UI State")] -> w351
          tunnel: w350 -> [w364 _]
          frame "Idle", Default {
            n140 = local read "List Number"() -> (w384:i32)
            n141 = local write "Stop"(0 ("Stop")) -> ()
            n142 = call "Run List.vi"("error in"=w383, "Numeric"=w384, "VISA resource name"=w380) -> ("error out"=w371:errorcluster)  [unwired: 7 in, 1 out]
            n143 = case shown="False" "Enable Logging" {
              tunnel: w382 -> [w406 w415]
              tunnel: "List Start" ("Message") -> [w401 w407]
              tunnel: [w405 w414] -> w368
              tunnel: w371 -> [w403 w412]
              tunnel: [w404 w409] -> w370
              tunnel: w364 -> [_ w408]
              frame False {
                n144 = call-poly "Enqueue Message.vi"("Priority Message? (F)"=TRUE, "error in (no error)"=w403, "Message"=w401, "Message Queue"=w406) -> ("error out"=w404:errorcluster, "dup Message Queue"=w405:refnum<queue>)  [unwired: 6 in]
              }
              frame True {
                n145 = call-poly "Enqueue Message.vi"("Priority Message? (F)"=TRUE, "error in (no error)"=w412, "Message"=w407, "Message Queue"=w415) -> ("error out"=w411:errorcluster, "dup Message Queue"=w414:refnum<queue>)  [unwired: 6 in]
                n146 = call-poly "Enqueue Message.vi"("Priority Message? (F)"=TRUE, "error in (no error)"=w412, "Message"=w407, "Message Queue"=w408) -> ("error out"=w410:errorcluster)  [unwired: 6 in, 1 out]
                n147 = Merge Errors(w411, w410) -> (w409:errorcluster)
              }
            }
            n148 = while {
              tunnel: [w420] -> w366
              tunnel: w370 -> [w420]
              stop <- w425 stop-if-true
              n149 = local read "Stop"() -> (w421:i32)
              n150 = Equal?(x=w421, y=40) -> (x = y?=w424:bool)
              n151 = Or(x=w424, y="Abort List") -> (x .or. y?=w425:bool)
            }
            n152 = local read "Enable Logging"() -> (w363:bool)
            n153 = case shown="False" w363 {
              tunnel: w368 -> [w390 w399]
              tunnel: "Stop" ("Message") -> [w385 w391]
              tunnel: [w389 w398] -> _
              tunnel: w366 -> [w387 w396]
              tunnel: [w388 w393] -> w362
              tunnel: w364 -> [_ w392]
              frame False {
                n154 = call-poly "Enqueue Message.vi"("Priority Message? (F)"=TRUE, "error in (no error)"=w387, "Message"=w385, "Message Queue"=w390) -> ("error out"=w388:errorcluster, "dup Message Queue"=w389:refnum<queue>)  [unwired: 6 in]
              }
              frame True {
                n155 = call-poly "Enqueue Message.vi"("Priority Message? (F)"=TRUE, "error in (no error)"=w396, "Message"=w391, "Message Queue"=w399) -> ("error out"=w395:errorcluster, "dup Message Queue"=w398:refnum<queue>)  [unwired: 6 in]
                n156 = call-poly "Enqueue Message.vi"("Priority Message? (F)"=TRUE, "error in (no error)"=w396, "Message"=w391, "Message Queue"=w392) -> ("error out"=w394:errorcluster)  [unwired: 6 in, 1 out]
                n157 = Merge Errors(w395, w394) -> (w393:errorcluster)
              }
            }
            n158 = call "List End.vi"("Output State"="Keep Output Enable", "error in"=w362, "VISA resource name"=w380) -> ("error out"=w379:errorcluster)  [unwired: 7 in, 1 out]
            n159 = flat-sequence {
              tunnel: [w419] -> w377
              tunnel: w378 -> [w419]
              tunnel: T11."Enabled" ("Disabled") -> [w418]
              tunnel: T11."Disabled and Grayed Out" ("Disabled") -> [w417]
              frame #0 {
                n160 = property on="Run List" class="Bool"("DisabledEnum"=w418) -> ()  [unwired: 2 in, 2 out]
                n161 = property on="Abort List" class="Bool"("DisabledEnum"=w417) -> ()  [unwired: 2 in, 2 out]
              }
            }
            n162 = call-poly "Enqueue Message.vi"("error in (no error)"=w379, "Message Data"="List Run Complete", "Message"="Update Status", "Message Queue"=w365) -> ("error out"=w378:errorcluster)  [unwired: 6 in, 1 out]
          }
          frame "Acquiring and Logging" {
            # "Stop Data acquire and logging before proceeding with running a list. This prevents timing issues."
            n163 = call-poly "Enqueue Message.vi"("Priority Message? (F)"=TRUE, "error in (no error)"=w430, "Message"="Stop", "Message Queue"=w431) -> ("error out"=w433:errorcluster)  [unwired: 6 in, 1 out]
            n164 = call-poly "Enqueue Message.vi"("error in (no error)"=w433, "Message"="Run List", "Message Queue"=w426) -> ("error out"=w428:errorcluster)  [unwired: 7 in, 1 out]
            n165 = One Button Dialog(message="Acquisition and Logging will stopped\nwill briefly stop in order to enable list mode.") -> ()  [unwired: 1 in, 1 out]
          }
        }
      }
      frame "External List" {
        # "Run the set external program. Note there is overhead for the command write times. All readings are done in the Acquisition Message loop. The  elapse time does not include the write time."
        n166 = Unbundle By Name(w443) -> ("Hardware Configuration.VISA resource name"=w436:refnum<visa-resource-name>)
        n167 = case shown="\"Idle\", Default" w439 {
          tunnel: [UI_State."Idle" ("UI State") UI_State."Idle" ("UI State")] -> w442
          tunnel: w441 -> [w452 w510]
          tunnel: [w449 w509] -> w440
          tunnel: w436 -> [w447 _]
          tunnel: w438 -> [_ w512]
          tunnel: w437 -> [_ w511]
          tunnel: w436 -> [w446 _]
          frame "Idle", Default {
            n168 = while {
              tunnel: w446 -> [w467]
              tunnel: w452 -> [w466]
              tunnel: [w465] -> w451
              i -> [w463]
              stop <- w461 stop-if-true
              n169 = local read "List Repeat"() -> (w459:i32)
              n170 = Increment(x=w463) -> (x+1=w460:i32)
              n171 = Array Size(array="Ext. List Array") -> (size(s)=w458:i32)
              n172 = while {
                tunnel: w467 -> [w489]
                tunnel: w466 -> [w488]
                tunnel: [w472] -> w465
                tunnel: "Ext. List Array" -> [w487] mode=indexing
                tunnel: w460 -> [_]
                tunnel: w459 -> [w485]
                tunnel: w458 -> [w481]
                tunnel: ["Ext. List Abort"] -> w457
                i -> [w486]
                stop <- w480 stop-if-true
                n173 = local read "Current Step"() -> (w476:i32)
                n174 = Unbundle(w487) -> ("Boolean"=w492:bool, "Ext. List Time"=w471:dbl, "Ext. List Current"=w491:dbl, "Ext. List Voltage"=w490:dbl)
                n175 = Increment(x=w486) -> (x+1=w478:i32)
                n176 = call <instrlib>:"Configure Output.vi"("Enable Output (T: Enable)"=w492, "error in (no error)"=w488, "Voltage Level (0.0 V)"=w490, "Address (0)"=w491, "VISA resource name"=w489) -> ("error out"=w475:errorcluster)  [unwired: 5 in, 1 out]
                n177 = Multiply(x=w481, y=w485) -> (x*y=w483:i32)
                n178 = call <vilib>:"High Resolution Relative Seconds.vi"() -> ("relative seconds"=w473:dbl)
                n179 = Increment(x=w476) -> (x+1=w477:i32)
                n180 = Subtract(x=w483, y=w477) -> (x-y=w484:i32)
                n181 = flat-sequence {
                  tunnel: w473 -> [w497]
                  tunnel: [w495] -> w469
                  tunnel: [w494] -> w468
                  tunnel: [w493] -> w474
                  tunnel: w475 -> [w493]
                  frame #0 {
                    n182 = local read "Delay Time"() -> (w494:dbl)
                    n183 = call <vilib>:"High Resolution Relative Seconds.vi"() -> ("relative seconds"=w496:dbl)
                    n184 = Subtract(x=w496, y=w497) -> (x-y=w495:dbl)
                  }
                }
                n185 = Equal?(x=w481, y=w478) -> (x = y?=w482:bool)
                n186 = local write "Current Step"(w477) -> ()
                n187 = local write "Remaining Steps"(w484) -> ()
                n188 = Or(x=w482, y="Ext. List Abort") -> (x .or. y?=w480:bool)
                n189 = Add(x=w469, y=w468) -> (x+y=→"Delay Time":dbl)
                n190 = call <vilib>:"High Resolution Polling Wait.vi"("error in (no error)"=w474, "seconds to wait"=w471) -> ("error out"=w472:errorcluster)  [unwired: 9 in]
              }
              n191 = Equal?(x=w459, y=w460) -> (x = y?=w462:bool)
              n192 = Compound Arithmetic op=OR(w457, w462) -> (w461:bool)
            }
            n193 = Get Date/Time In Seconds() -> (seconds since 1Jan1904=w454:timestamp)
            n194 = call <vilib>:"High Resolution Relative Seconds.vi"() -> ("relative seconds"=w455:dbl)
            n195 = Format Date/Time String(seconds (now)=w454) -> (date/time string=→"Start Time":string)  [unwired: 2 in]
            n196 = flat-sequence {
              tunnel: w451 -> [w507]
              tunnel: [w507] -> w450
              tunnel: w455 -> [w506]
              frame #0 {
                n197 = Get Date/Time In Seconds() -> (seconds since 1Jan1904=w505:timestamp)
                n198 = local read "Delay Time"() -> (w502:dbl)
                n199 = call <vilib>:"High Resolution Relative Seconds.vi"() -> ("relative seconds"=w503:dbl)
                n200 = property on="Ext. List Abort" class="Bool"("DisabledEnum"=2) -> ()  [unwired: 2 in, 2 out]
                n201 = Subtract(x=w503, y=w506) -> (x-y=w501:dbl)
                n202 = Format Date/Time String(seconds (now)=w505) -> (date/time string=→"Stop Time":string)  [unwired: 2 in]
                n203 = Subtract(x=w501, y=w502) -> (x-y=→"Elapsed Time (s)":dbl)
                n204 = property on="Ext. List Start" class="Bool"("DisabledEnum"=0) -> ()  [unwired: 2 in, 2 out]
              }
            }
            n205 = local write "Delay Time"(0.0 ("Delay Time")) -> ()
            n206 = call <instrlib>:"Enable Output.vi"("error in (no error)"=w450, "Enable Output (F: False)"=FALSE, "VISA resource name"=w447) -> ("error out"=w449:errorcluster)  [unwired: 7 in, 1 out]
          }
          frame "Acquiring and Logging" {
            # "Stop Data acquire and logging before proceeding with running a list. This prevents timing issues. Logging and external function can be added by adding a case in Acquisition Message Loop.vi However the timing of each step will be less accurate since overhead for each read would have to be included."
            n207 = call-poly "Enqueue Message.vi"("Priority Message? (F)"=TRUE, "error in (no error)"=w510, "Message"="Stop", "Message Queue"=w511) -> ("error out"=w515:errorcluster)  [unwired: 6 in, 1 out]
            n208 = call-poly "Enqueue Message.vi"("error in (no error)"=w515, "Message"="External List", "Message Queue"=w512) -> ("error out"=w509:errorcluster)  [unwired: 7 in, 1 out]
            n209 = One Button Dialog(message="Acquisition and Logging will stopped\nwill briefly stop in order to enable list mode.") -> ()  [unwired: 1 in, 1 out]
          }
        }
      }
      frame "Start" {
        # "Message Acquisition and Logging loops to start."
        # "Enable: Stop\nDisable: Start, Exit, Settings"
        # "Start - Enable/Disable buttons appropriately for an acquisition that has started, and update status display."
        n210 = Unbundle By Name(w536) -> ("Stop Ref"=w531:refnum<vi>, "Start Ref"=w530:refnum<vi>, "Exit Ref"=w529:refnum<vi>, "Connect Ref"=w528:refnum<vi>)
        n211 = Build Array(w530, w529, w528) -> (w534:refnum<vi>[])
        n212 = Build Array(w531) -> (w533:refnum<vi>[])
        n213 = call "Set Enable State on Multiple Controls.vi"("Enable?"=FALSE, "Controls"=w534) -> ()  [unwired: 10 in]
        n214 = call "Set Enable State on Multiple Controls.vi"("Enable?"=TRUE, "Controls"=w533) -> ()  [unwired: 10 in]
        n215 = call-poly "Enqueue Message.vi"("error in (no error)"=w518, "Message Data"="Acquiring and Logging..." ("Acquiring and Logging..."), "Message"="Update Status", "Message Queue"=w519) -> ("error out"=w527:errorcluster)  [unwired: 6 in, 1 out]
        n216 = call-poly "Enqueue Message.vi"("error in (no error)"=w527, "Message"="Start", "Message Queue"=w520) -> ("error out"=w525:errorcluster)  [unwired: 7 in, 1 out]
        n217 = call-poly "Enqueue Message.vi"("error in (no error)"=w525, "Message"="Start", "Message Queue"=w523) -> ("error out"=w524:errorcluster)  [unwired: 7 in, 1 out]
      }
      frame "Stop" {
        w542 = TRUE ("Priority Message? (F)")
        # "Message Acquisition and Logging loops to stop"
        # "Enable: Start, Exit, Settings\nDisable: Stop"
        # "Stop - Enable/Disable buttons appropriately for an acquisition that has stopped, and update status display."
        n218 = Unbundle By Name(w558) -> ("Stop Ref"=w553:refnum<vi>, "Start Ref"=w552:refnum<vi>, "Exit Ref"=w551:refnum<vi>, "Connect Ref"=w550:refnum<vi>)
        n219 = Build Array(w552, w551, w550) -> (w556:refnum<vi>[])
        n220 = Build Array(w553) -> (w555:refnum<vi>[])
        n221 = call "Set Enable State on Multiple Controls.vi"("Enable?"=TRUE, "Controls"=w556) -> ()  [unwired: 10 in]
        n222 = call "Set Enable State on Multiple Controls.vi"("Enable?"=FALSE, "Controls"=w555) -> ()  [unwired: 10 in]
        n223 = call-poly "Enqueue Message.vi"("Priority Message? (F)"=w542, "error in (no error)"=w540, "Message"="Stop", "Message Queue"=w548) -> ("error out"=w544:errorcluster)  [unwired: 6 in, 1 out]
        n224 = call-poly "Enqueue Message.vi"("Priority Message? (F)"=w542, "error in (no error)"=w544, "Message"="Stop", "Message Queue"=w541) -> ("error out"=w543:errorcluster)  [unwired: 6 in, 1 out]
        n225 = case shown="Default" w545 {
          selector: w545 -> [w560 _]
          tunnel: [w560 UI_State."Waiting for Stop" ("UI State")] -> w546
          frame "Waiting for Exit" {
          }
          frame Default {
          }
        }
      }
      frame "Acquisition Stopped" {
        # "Logic for determining what action to take when the acquisition has stopped."
        n226 = case shown="Default" w566 {
          selector: w566 -> [w570 _ _ _ _]
          tunnel: w565 -> [w569 w572 w574 w580 w586]
          tunnel: w564 -> [_ _ _ w578 w583]
          tunnel: [w570 UI_State."Waiting for Exit (Acq Stopped)" ("UI State") UI_State."Waiting for Stop (Acq Stopped)" ("UI State") UI_State."Idle" ("UI State") UI_State."Idle" ("UI State")] -> w563
          tunnel: [w569 w572 w574 w579 w584] -> w562
          frame Default {
          }
          frame "Waiting for Exit", "Waiting for Exit (Acq Stopped)" {
          }
          frame "Waiting for Stop", "Waiting for Stop (Acq Stopped)" {
          }
          frame "Waiting for Exit (Log Stopped)" {
            # "If we are waiting to exit, and the logging has already stopped, then the \"Acquisition Stopped\" message indicates that it is time to exit."
            n227 = call-poly "Enqueue Message.vi"("Priority Message? (F)"=TRUE, "error in (no error)"=w580, "Message"="Exit", "Message Queue"=w578) -> ("error out"=w579:errorcluster)  [unwired: 6 in, 1 out]
          }
          frame "Waiting for Stop (Log Stopped)" {
            # "If we are waiting to stop, and the logging has already stopped, then the \"Acquisition Stopped\" message indicates that it is time to stop."
            n228 = call-poly "Enqueue Message.vi"("error in (no error)"=w586, "Message Data"="Ready..." ("Ready..."), "Message"="Update Status", "Message Queue"=w583) -> ("error out"=w584:errorcluster)  [unwired: 6 in, 1 out]
          }
        }
      }
      frame "Logging Stopped" {
        # "Logic for determining what action to take when the logging has stopped."
        n229 = case shown="\"Waiting for Stop (Acq Stopped)\"" w591 {
          selector: w591 -> [w595 _ _ _ _]
          tunnel: w590 -> [w594 w597 w599 w605 w608]
          tunnel: w589 -> [_ _ _ w603 w607]
          tunnel: [w595 UI_State."Waiting for Exit (Log Stopped)" ("UI State") UI_State."Waiting for Stop (Log Stopped)" ("UI State") UI_State."Idle" ("UI State") UI_State."Idle" ("UI State")] -> w588
          tunnel: [w594 w597 w599 w604 w606] -> w587
          frame Default {
          }
          frame "Waiting for Exit", "Waiting for Exit (Log Stopped)" {
          }
          frame "Waiting for Stop", "Waiting for Stop (Log Stopped)" {
          }
          frame "Waiting for Exit (Acq Stopped)" {
            # "If we are waiting to exit, and the acquisition has already stopped, then the \"Logging Stopped\" message indicates that it is time to exit."
            n230 = call-poly "Enqueue Message.vi"("Priority Message? (F)"=TRUE, "error in (no error)"=w605, "Message"="Exit", "Message Queue"=w603) -> ("error out"=w604:errorcluster)  [unwired: 6 in, 1 out]
          }
          frame "Waiting for Stop (Acq Stopped)" {
            # "If we are waiting to stop, and the acquisition has already stopped, then the \"Logging Stopped\" message indicates that it is time to stop."
            n231 = call-poly "Enqueue Message.vi"("error in (no error)"=w608, "Message Data"="Ready..." ("Ready..."), "Message"="Update Status", "Message Queue"=w607) -> ("error out"=w606:errorcluster)  [unwired: 6 in, 1 out]
          }
        }
      }
      frame "Broadcast settings" {
        w617 = "Update Settings" ("Message")
        # "Broadcast settings - Send the 'Update Settings' message to the Logging and Acquisition message loops."
        n232 = Unbundle By Name(w622) -> ("Hardware Configuration"=w621:T8, "Logging Configuration"=w620:T9)
        n233 = call-poly "Enqueue Message.vi"("Message Data"=w621, "Message"=w617, "Message Queue"=w615) -> ("error out"=w623:errorcluster)  [unwired: 7 in, 1 out]
        n234 = call-poly "Enqueue Message.vi"("error in (no error)"=w623, "Message Data"=w620, "Message"=w617, "Message Queue"=w614) -> ("error out"=w619:errorcluster)  [unwired: 6 in, 1 out]
        n235 = Merge Errors(w619, w618) -> (w612:errorcluster)
      }
      frame "Launch Settings Dialog" {
        # "Launch Settings Dialog - Launch the Settings Dialog when corresponding button is presset. \nInst. Settings, PS Settings, or Log Settings"
        n236 = local read "Settings CtlRef"() -> (w628:refnum<vi>)
        n237 = property on="Property Node" class="Bool"(reference=w628) -> ("Label.Text"=w626:string)  [unwired: 1 in, 2 out]
        n238 = case shown="\"Log Settings\"" w626 {
          tunnel: w632 -> [w634 w642 w657 w669]
          tunnel: [w634 w639 w652 w672] -> w629
          tunnel: w627 -> [_ w638 w655 w667]
          tunnel: w625 -> [w633 w637 w658 w671]
          tunnel: [w633 w635 w650 w666] -> w624
          frame "False", Default {
          }
          frame "Inst. Settings" {
            n239 = call-by-ref "?"("error in (no error)"=w642, "Settings in"=w637) -> ("error out"=w640:errorcluster, "Cancelled?"=w641:bool, "Settings out"=w636:T7)  [unwired: 8 in, 3 out]
            n240 = case shown="False" w641 {
              tunnel: w638 -> [w647 _]
              tunnel: w640 -> [w646 w649]
              tunnel: [w645 w649] -> w639
              tunnel: w636 -> [w643 w648]
              tunnel: [w643 w648] -> w635
              frame False {
                n241 = call-poly "Enqueue Message.vi"("error in (no error)"=w646, "Message"="Broadcast Settings", "Message Queue"=w647) -> ("error out"=w645:errorcluster)  [unwired: 7 in, 1 out]
              }
              frame True {
              }
            }
          }
          frame "PS Settings" {
            n242 = local read "model"() -> (w651:string)
            n243 = call-by-ref "?"("error in"=w657, "Model"=w651, "Settings in"=w658) -> ("error out"=w656:errorcluster, "Cancelled?"=w654:bool, "Settings out"=w653:T7)  [unwired: 7 in, 3 out]
            n244 = case shown="False" w654 {
              tunnel: w655 -> [w663 _]
              tunnel: w656 -> [w662 w665]
              tunnel: [w661 w665] -> w652
              tunnel: [w659 w664] -> w650
              tunnel: w653 -> [w659 w664]
              frame False {
                n245 = call-poly "Enqueue Message.vi"("error in (no error)"=w662, "Message"="Config PS Settings", "Message Queue"=w663) -> ("error out"=w661:errorcluster)  [unwired: 7 in, 1 out]
              }
              frame True {
              }
            }
          }
          frame "Log Settings" {
            n246 = call-by-ref "?"("error in (no error)"=w669, "Settings in"=w671) -> ("error out"=w668:errorcluster, "Cancelled?"=w673:bool, "Settings out"=w670:T7)  [unwired: 8 in, 3 out]
            n247 = case shown="False" w673 {
              tunnel: w667 -> [w678 _]
              tunnel: w668 -> [w677 w680]
              tunnel: [w676 w680] -> w672
              tunnel: [w674 w679] -> w666
              tunnel: w670 -> [w674 w679]
              frame False {
                n248 = call-poly "Enqueue Message.vi"("error in (no error)"=w677, "Message"="Broadcast Settings", "Message Queue"=w678) -> ("error out"=w676:errorcluster)  [unwired: 7 in, 1 out]
              }
              frame True {
              }
            }
          }
        }
      }
      frame "Config PS Settings" {
        # "Current \nLimit"
        # "Voltage Limit \nProtection Delay"
        # "Max/MIN\nVoltage"
        # "Configure the instruments output parameters."
        n249 = Unbundle By Name(w696) -> ("Current Limit"=w681:dbl, "OVP State"=w684:bool, "OVP Limit"=w683:dbl, "OVP Delay"=w682:dbl, "Voltage Limit"=w695:cluster{"Numeric":dbl, "Numeric":dbl}, "Hardware Configuration.VISA resource name"=w694:refnum<visa-resource-name>)
        n250 = Unbundle(w695) -> ("Numeric"=w686:dbl, "Numeric"=w685:dbl)
        n251 = call <instrlib>:"Configure Voltage Limit.vi"("VISA resource name"=w694, "Max Voltage Limit (80.000 V)"=w686, "Min Voltage Limit (0.000 V)"=w685, "error in (no error)"=w688) -> ("VISA resource name out"=w691:refnum<visa-resource-name>, "error out"=w692:errorcluster)  [unwired: 10 in]
        n252 = call <instrlib>:"Configure OVP.vi"("VISA resource name"=w691, "Enable OVP (T: Enable)"=w684, "Voltage Limit (80.000 V)"=w683, "Protection Delay (0.001)"=w682, "error in (no error)"=w692) -> ("VISA resource name out"=w690:refnum<visa-resource-name>, "error out"=w693:errorcluster)  [unwired: 9 in]
        n253 = call <instrlib>:"Configure Current Limit.vi"("error in (no error)"=w693, "Current Limit (0.0 A)"=w681, "VISA resource name"=w690) -> ("error out"=w689:errorcluster)  [unwired: 7 in, 1 out]
      }
      frame "Error" {
        # "Error - Display an error dialog. This message is sent by the \"Error Handler\" VIs at the end of other loops in this application."
        n254 = Variant To Data(error in=w698, type=errorcluster {"status"=FALSE, "code"=0, "source"=""} ("error constant"), Variant=w701) -> (data=w699:errorcluster, error out=w702:errorcluster)
        n255 = call <vilib>:"Simple Error Handler.vi"("error in (no error)"=w699) -> ()  [unwired: 4 in, 5 out]
      }
      frame "Confirm Quit" {
        # "Confirm Quit - Message that can confirm whether or not the user wants to exit the application."
        n256 = case shown="\"Acquiring and Logging\"" w710 {
          tunnel: w709 -> [w718 w722]
          tunnel: w708 -> [w717 w721]
          tunnel: [w716 w720] -> w707
          tunnel: [UI_State."Idle" ("UI State") w719] -> w706
          frame Default {
            # "If 'Confirm Quit' comes in while the system is idle, there is no need for a confirmation message."
            n257 = call-poly "Enqueue Message.vi"("Priority Message? (F)"=TRUE, "error in (no error)"=w717, "Message"="Exit", "Message Queue"=w718) -> ("error out"=w716:errorcluster)  [unwired: 6 in, 1 out]
          }
          frame "Acquiring and Logging" {
            n258 = Two Button Dialog(message="Are you sure you want to quit while the acquisition is running?" ("Confirm Quit Message"), 1:"No" ("No"), 2:"Yes" ("Yes")) -> (T button?=w723:bool)
            n259 = case shown="True" w723 {
              tunnel: w722 -> [_ w732]
              tunnel: w721 -> [w728 w733]
              tunnel: [w728 w731] -> w720
              tunnel: [UI_State."Acquiring and Logging" ("UI State") UI_State."Waiting for Exit" ("UI State")] -> w719
              frame False {
                # "User did not want to quit."
              }
              frame True {
                n260 = call-poly "Enqueue Message.vi"("error in (no error)"=w733, "Message"="Stop", "Message Queue"=w732) -> ("error out"=w731:errorcluster)  [unwired: 7 in, 1 out]
              }
            }
          }
        }
      }
      frame "Disconnect" {
        # "Disconnects the instrument, closes the session and reinitializes the UI."
        n261 = Unbundle By Name(w739) -> ("Hardware Configuration.VISA resource name"=w738:refnum<visa-resource-name>)
        n262 = call-poly "Enqueue Message.vi"("error in (no error)"=w737, "Message"="Init UI Refs", "Message Queue"=w735) -> ("error out"=w736:errorcluster)  [unwired: 7 in, 1 out]
        n263 = call <instrlib>:"Close.vi"("error in (no error)"=w736, "VISA resource name"=w738) -> ("error out"=w740:errorcluster)  [unwired: 9 in]
      }
      frame "Exit" {
        w748 = TRUE ("Priority Message? (F)")
        w749 = "Exit" ("Message")
        # "Popup an error dialog if 'Exit' was called as a result of an error."
        # "Stop the VI"
        # "Exit - Send Exit messages to the Acquisition and Logging loops, and fire the user event to stop the Event Handling Loop."
        n264 = Variant To Data(type=errorcluster {"status"=FALSE, "code"=0, "source"=""} ("error constant"), Variant=w744) -> (data=w743:errorcluster)  [unwired: 1 in, 1 out]
        n265 = call <vilib>:"Simple Error Handler.vi"("error in (no error)"=w743) -> ()  [unwired: 4 in, 5 out]
        n266 = call-poly "Enqueue Message.vi"("Priority Message? (F)"=w748, "error in (no error)"=w746, "Message"=w749, "Message Queue"=w753) -> ("error out"=w750:errorcluster)  [unwired: 6 in, 1 out]
        n267 = call-poly "Enqueue Message.vi"("Priority Message? (F)"=w748, "error in (no error)"=w750, "Message"=w749, "Message Queue"=w752) -> ("error out"=w747:errorcluster)  [unwired: 6 in, 1 out]
        n268 = call "Fire User Event - Stop.vi"("error in (no error)"=w747, "User Event - Stop"=w757) -> ("error out"=w756:errorcluster)  [unwired: 9 in]
      }
      frame "---Copy This Frame---" {
        # "Duplicate this frame when creating new messages.  Change this comment in the duplicated frame to describe this message."
        n269 = Merge Errors(w763) -> (w762:errorcluster)
      }
      frame Default {
        # "'Default' case only runs if there is a message that isn't defined in any of the other cases.  Output a programming error."
        n270 = xnode "Error Ring"("parameter 0"=w765) -> ("error out"=w764:errorcluster)
      }
    }
    n271 = call "Error Handler - Message Handling Loop.vi"("error in (no error)"=w42, "Message Queue"=w41) -> ("dup error in"=w43:errorcluster)  [unwired: 8 in, 1 out]
    "UI State" <- w39
  }
  n272 = while {
    tunnel: w17 -> [w781]
    tunnel: [w778] -> w31
    shift-right: [w780] -> w23
    shift-left: w13 -> [w782]
    stop <- w779 stop-if-true
    # "Event Handling Loop"
    n273 = event shown="[14] <User Event - Stop>: User Event" {
      selector: w782 -> [_ _ _ _ _ _ _ _ _ _ _ _ _ _ _]
      dyn-events: [_ _ _ _ _ _ _ _ _ _ _ _ _ _ _] -> w780
      timeout: _ -> [_ _ _ _ _ _ _ _ _ _ _ _ _ _ _]
      tunnel: [_ _ _ _ _ _ _ _ _ _ _ _ _ _ TRUE ("Discard?")] -> w779
      tunnel: w781 -> [w786 w787 w811 w817 w820 w824 w831 w835 w848 w851 w856 w859 w861 w870 w871]
      tunnel: [w784 w789 _ w815 _ w826 w828 w833 _ w850 w854 _ w864 w868 _] -> w777
      tunnel: [w783 w790 w810 w816 w820 w827 w830 w834 w847 w849 w855 w859 w860 w869 w871] -> w776
      event "Start": Value Change {
        n274 = event-data() -> ()  [unwired: 1 in, 1 out]
        n275 = call-poly "Enqueue Message.vi"("Message"="Start", "Message Queue"=w786) -> ("error out"=w784:errorcluster, "dup Message Queue"=w783:refnum<queue>)  [unwired: 8 in]
      }
      event Menu Selection (User) {
        n276 = event-data() -> ("ItemTag"=w788:string)  [unwired: 1 in]
        n277 = case shown="\"Help Guide\"" w788 {
          tunnel: [w792 w794 w795] -> w790
          tunnel: w787 -> [w792 w794 w795]
          tunnel: [errorcluster {"status"=FALSE, "code"=0, "source"=""} ("error out") w793 w799] -> w789
          frame "False", Default {
          }
          frame "About" {
            n278 = call-by-ref "?"() -> (error out=w793:errorcluster)  [unwired: 14 in, 1 out]
          }
          frame "Help Guide" {
            n279 = call <vilib>:"Application Directory.vi"() -> ("Application Directory"=w796:path)
            n280 = Build Path(base path=w796, name or relative path=path "data/Help.pdf") -> (appended path=w807:path)
            n281 = Path To String(path=w807) -> (string=w805:string)
            n282 = Search and Replace String(replace all?=TRUE ("replace all? (F)"), input string=w805, search string="\\", replace string="/" ("replace string (\"\")")) -> (result string=w802:string, error out=w800:errorcluster)  [unwired: 4 in, 2 out]
            n283 = Format Into String(format string="file:///%s" ("URL"), error in=w800, w802) -> (resulting string=w808:string, error out=w801:errorcluster)  [unwired: 1 in]
            n284 = call-poly <vilib>:"Open URL in Default Browser.vi"("error in (no error)"=w801, "URL"=w808) -> ("error out"=w799:errorcluster)  [unwired: 4 in, 1 out]
          }
        }
      }
      event "Inst. Settings", "PS Settings", "Log Settings": Value Change {
        n285 = event-data() -> ("CtlRef"=→"Settings CtlRef":refnum<vi>)  [unwired: 1 in]
        n286 = call-poly "Enqueue Message.vi"("Message"="Launch Settings Dialog", "Message Queue"=w811) -> ("dup Message Queue"=w810:refnum<queue>)  [unwired: 8 in, 1 out]
      }
      event "Connect": Value Change {
        n287 = event-data() -> ()  [unwired: 1 in, 1 out]
        n288 = call-poly "Enqueue Message.vi"("Message"="Init INST", "Message Queue"=w817) -> ("error out"=w815:errorcluster, "dup Message Queue"=w816:refnum<queue>)  [unwired: 8 in]
        n289 = property on="Disconnect" class="Bool"("DisabledEnum"=T11."Enabled" ("Disabled")) -> ()  [unwired: 2 in, 2 out]
        n290 = property on="Connect" class="Bool"("DisabledEnum"=T11."Disabled and Grayed Out" ("Disabled")) -> ()  [unwired: 2 in, 2 out]
      }
      event "Clear": Value Change {
        w819 = dbl[] [] ("History Data")
        # "Clears all data for the 3 monitoring charts."
        n291 = event-data() -> ()  [unwired: 1 in, 1 out]
        n292 = property on="Voltage" class="WFChart (strict)"("History Data"=w819) -> ()  [unwired: 2 in, 2 out]
        n293 = property on="Current" class="WFChart (strict)"("History Data"=w819) -> ()  [unwired: 2 in, 2 out]
        n294 = property on="Power" class="WFChart (strict)"("History Data"=w819) -> ()  [unwired: 2 in, 2 out]
      }
      event "Voltage", "Current", "Output Control": Value Change {
        n295 = event-data() -> ("CtlRef"=→"Output Ref":refnum<vi>)  [unwired: 1 in, 2 out]
        n296 = Flush Queue(queue=w824) -> (queue out=w823:refnum<queue>, error out=w822:errorcluster)  [unwired: 1 in, 1 out]
        n297 = call "Enqueue to Front Message (Single).vi"("error in (no error)"=w822, "Message"="Output Param Config", "Message Queue"=w823) -> ("error out"=w826:errorcluster, "dup Message Queue"=w827:refnum<queue>)  [unwired: 7 in]
      }
      event "Save Sequence to PS", "Load Sequence from PS", "Save List to PS", "Load List from PS": Value Change {
        n298 = event-data() -> ("CtlRef"=→"List CtlRef":refnum<vi>)  [unwired: 1 in]
        n299 = call-poly "Enqueue Message.vi"("Message"="List Action", "Message Queue"=w831) -> ("error out"=w828:errorcluster, "dup Message Queue"=w830:refnum<queue>)  [unwired: 8 in]
      }
      event "Run List": Value Change {
        (unwired) TRUE
        n300 = event-data() -> ()  [unwired: 1 in, 1 out]
        n301 = call-poly "Enqueue Message.vi"("Message Data"="Running List " ("Acquiring and Logging..."), "Message"="Update Status", "Message Queue"=w835) -> ("error out"=w838:errorcluster, "dup Message Queue"=w839:refnum<queue>)  [unwired: 7 in]
        n302 = call-poly "Enqueue Message.vi"("error in (no error)"=w838, "Message"="Run List", "Message Queue"=w839) -> ("error out"=w833:errorcluster, "dup Message Queue"=w834:refnum<queue>)  [unwired: 7 in]
        n303 = property on="Run List" class="Bool"("DisabledEnum"=T11."Disabled and Grayed Out" ("Disabled")) -> ()  [unwired: 2 in, 2 out]
        n304 = property on="Abort List" class="Bool"("DisabledEnum"=T11."Enabled" ("Disabled")) -> ()  [unwired: 2 in, 2 out]
      }
      event "Ext. List Start": Value Change {
        n305 = event-data() -> ()  [unwired: 1 in, 1 out]
        n306 = call-poly "Enqueue Message.vi"("Message"="External List", "Message Queue"=w848) -> ("dup Message Queue"=w847:refnum<queue>)  [unwired: 8 in, 1 out]
        n307 = property on="Ext. List Start" class="Bool"("DisabledEnum"=T11."Disabled and Grayed Out" ("Disabled")) -> ()  [unwired: 2 in, 2 out]
        n308 = property on="Ext. List Abort" class="Bool"("DisabledEnum"=T11."Enabled" ("Disabled")) -> ()  [unwired: 2 in, 2 out]
        "Current Step" <- 0 ("Current Step")
      }
      event "Stop": Value Change {
        n309 = event-data() -> ()  [unwired: 1 in, 1 out]
        n310 = call-poly "Enqueue Message.vi"("Message"="Stop", "Message Queue"=w851) -> ("error out"=w850:errorcluster, "dup Message Queue"=w849:refnum<queue>)  [unwired: 8 in]
      }
      event Panel Close? {
        # "Send the 'Confirm Quit' message if the user closes the panel of the VI. Discard the event so the 'Confirm Quit' message has a chance to run."
        n311 = event-data() -> ()  [unwired: 1 in, 1 out]
        n312 = call-poly "Enqueue Message.vi"("Priority Message? (F)"=TRUE, "Message"="Confirm Quit", "Message Queue"=w856) -> ("error out"=w854:errorcluster, "dup Message Queue"=w855:refnum<queue>)  [unwired: 7 in]
        n313 = event-data("Discard?"=TRUE) -> ()  [unwired: 1 in, 1 out]
      }
      event Application Instance Close {
        n314 = event-data() -> ()  [unwired: 1 in, 1 out]
      }
      event "Exit": Value Change {
        w862 = TRUE  # Priority Message
        # "The UI Message Loop handles sending the Exit message to other loops."
        n315 = event-data() -> ()  [unwired: 1 in, 1 out]
        n316 = call-poly "Enqueue Message.vi"("Priority Message? (F)"=w862, "Message"="Exit", "Message Queue"=w861) -> ("error out"=w864:errorcluster, "dup Message Queue"=w860:refnum<queue>)  [unwired: 7 in]
      }
      event "Disconnect": Value Change {
        w865 = T11."Enabled" ("Disabled")
        n317 = event-data() -> ()  [unwired: 1 in, 1 out]
        n318 = call-poly "Enqueue Message.vi"("Message"="Disconnect", "Message Queue"=w870) -> ("error out"=w868:errorcluster, "dup Message Queue"=w869:refnum<queue>)  [unwired: 8 in]
        n319 = property on="Disconnect" class="Bool"("DisabledEnum"=T11."Disabled and Grayed Out" ("Disabled")) -> ()  [unwired: 2 in, 2 out]
        n320 = property on="Connect" class="Bool"("DisabledEnum"=w865) -> ()  [unwired: 2 in, 2 out]
        n321 = property on="Inst. Settings" class="Bool"("DisabledEnum"=w865) -> ()  [unwired: 2 in, 2 out]
      }
      event User Event {
        # "The Message Handling Loop processed an \"Exit\" message, which fired this event to stop the Event Handling Loop."
        n322 = event-data() -> ()  [unwired: 1 in, 1 out]
        n323 = local write "Status"("Exit" ("Exit String")) -> ()
      }
    }
    n324 = call "Error Handler - Event Handling Loop.vi"("error in (no error)"=w777, "Message Queue"=w776) -> ("dup error in"=w778:errorcluster)  [unwired: 8 in, 1 out]
  }
  n325 = call "Logging Message Loop.vi"("error in (no error)"=w26, "Data Queue"=w9, "Message Queues"=w28) -> ("error out"=w27:errorcluster)  [unwired: 8 in]
  n326 = while "Data Display Loop" {
    tunnel: w1 -> [w880]
    stop <- w879 stop-if-true
    # "Voltage, Current Power Data Loop"
    n327 = Wait on Notification(notifier=w880) -> (notification=w878:T5, error out=w879:errorcluster)  [unwired: 3 in, 2 out]
    n328 = Unbundle By Name(w878) -> ("Voltage"=→"Voltage":dbl, "Current"=→"Current":dbl, "Power"=→"Power":dbl, "List Stop COND"=→"Stop":i32)
  }
  n329 = Release Queue(queue=w17, error in (no error)=w32) -> (error out=w15:errorcluster)  [unwired: 1 in, 2 out]
  n330 = Release Queue(queue=w9, error in (no error)=w15) -> (error out=w14:errorcluster)  [unwired: 1 in, 2 out]
  n331 = Unregister For Events(event registration refnum=w23, error in=w31) -> (error out=w24:errorcluster)
  n332 = Release Notifier(notifier=w2, error in (no error)=w14) -> (error out=w6:errorcluster)  [unwired: 1 in, 2 out]
  n333 = Release Notifier(notifier=w1, error in (no error)=w6) -> (error out=w5:errorcluster)  [unwired: 1 in, 2 out]
  n334 = Merge Errors(w24, w5, w30, w27) -> (w18:errorcluster)
  n335 = call "Destroy User Event - Stop.vi"("error in (no error)"=w18, "User Event - Stop"=w12) -> ("error out"=w16:errorcluster)  [unwired: 9 in]
  n336 = disable-structure shown="Default" {
    disable-tunnel: w16 -> [_ _]
    frame condition #0 (active) {
    }
    frame condition #1 {
      # "Call Quit LabVIEW if running as a built application."
      n337 = Quit LabVIEW() -> ()  [unwired: 1 in]
    }
  }
